vi "CAN Ref FGV.vi"(6 "CAN FGV State":T2=enum."Get", 8 "error in":errorcluster, 10 "Socket No":u16, 11 "object in":refnum<class "NI-XNET.lvclass">) -> (0 "error out":errorcluster, 2 "CAN Ref Data":T1, 3 "object out":refnum<class "NI-XNET.lvclass">)   [LabVIEW 2023, in "LTT_TeststandSteptypes.lvlib"]
uses:
  LTT_TeststandSteptypes.lvlib
  Control/CAN FGV State.ctl
  Control/CAN Ref Data.ctl
  HardwareAbstractionLayer_LVOOP/CAN/CAN Lib/NI-XNET_class/NI-XNET.lvclass
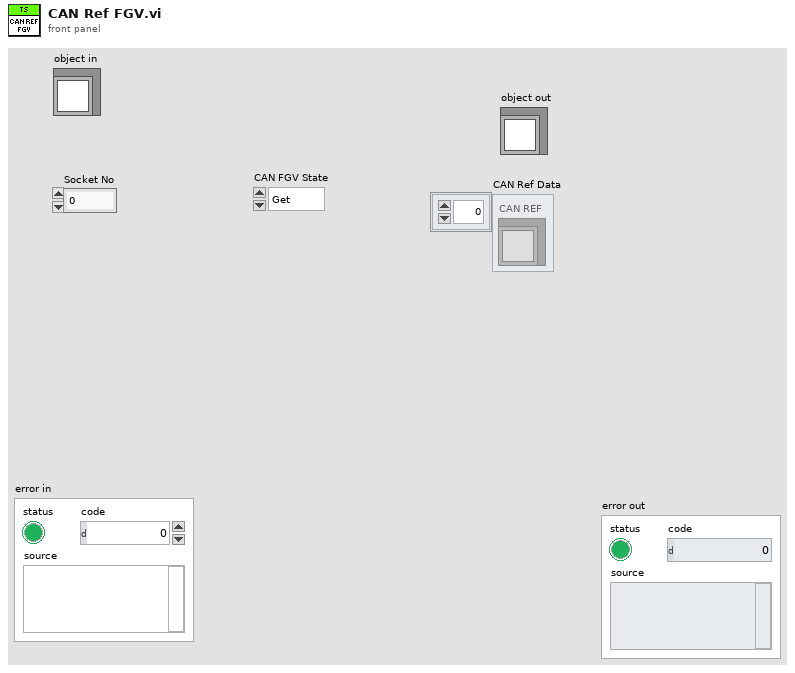
[diagram p1: front panel]
types:
  T1 = typedef "LTT_TeststandSteptypes.lvlib/CAN Ref Data.ctl" = refnum<class "NI-XNET.lvclass">[]
  T2 = typedef "LTT_TeststandSteptypes.lvlib/CAN FGV State.ctl" = enum16{"Init", "Get", "Set"}
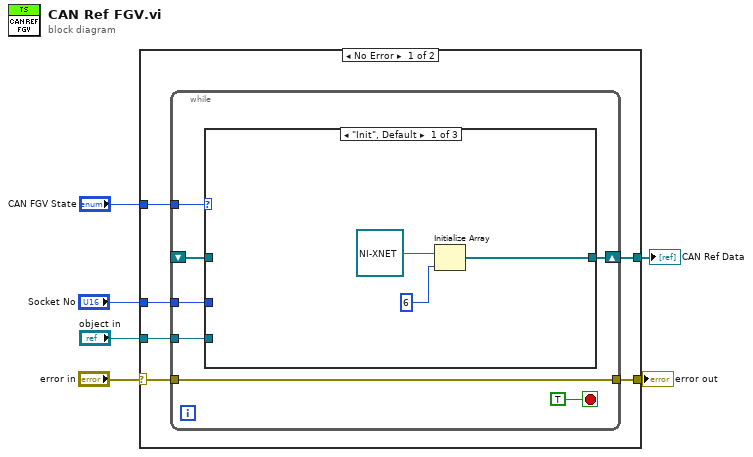
[diagram p0: block diagram]
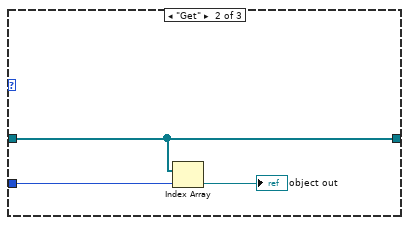
[diagram p2: hidden frame]
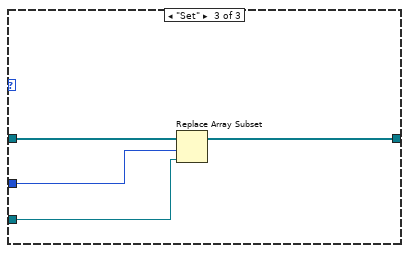
[diagram p3: hidden frame]
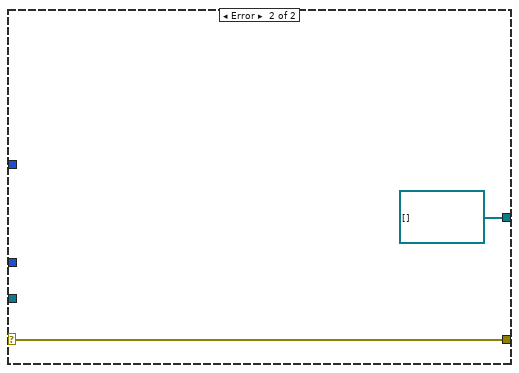
[diagram p4: hidden frame]
diagram:
  n1 = case shown="No Error" "error in" {
    selector: "error in" -> [w12 w31]
    tunnel: "CAN FGV State" -> [w11 _]
    tunnel: "object in" -> [w10 _]
    tunnel: "Socket No" -> [w9 _]
    tunnel: [w8 w31] -> w2
    tunnel: [w7 refnum<class "NI-XNET.lvclass">[] []] -> w1
    frame No Error {
      n2 = while {
        tunnel: w12 -> [w13]
        tunnel: w11 -> [w18]
        shift-right: [w17] -> w7
        shift-left: _ -> [w16]
        tunnel: w10 -> [w15]
        tunnel: w9 -> [w14]
        tunnel: [w13] -> w8
        stop <- TRUE stop-if-true
        n3 = case shown="\"Init\", Default" w18 {
          tunnel: [w22 w24 w28] -> w17
          tunnel: w16 -> [_ w24 w29]
          tunnel: w15 -> [_ _ w27]
          tunnel: w14 -> [_ w25 w26]
          frame "Init", Default {
            n4 = Initialize Array(refnum<class "NI-XNET.lvclass"> refnum ("object in"), 6 ("dimension size")) -> (w22:refnum<class "NI-XNET.lvclass">[])
          }
          frame "Get" {
            n5 = Index Array(array=w24, index=w25) -> (element=→"object out":refnum<class "NI-XNET.lvclass">)
          }
          frame "Set" {
            n6 = Replace Array Subset(array=w29, new element=w27, index=w26) -> (w28:refnum<class "NI-XNET.lvclass">[])
          }
        }
      }
    }
    frame Error {
    }
  }
  "error out" <- w2
  "CAN Ref Data" <- w1
